vi "WMP Init.vi"(8 "error in (no error)":errorcluster, 11 "Main Panel in":refnum<class "Main Panel.lvclass">) -> (0 "error out":errorcluster, 3 "Main Panel out":refnum<class "Main Panel.lvclass">)   [LabVIEW 2018, in "Main Panel.lvlib" / "Main Panel.lvclass"]
uses:
  Main Panel.lvclass
  Main Panel.lvclass/Main Panel.ctl
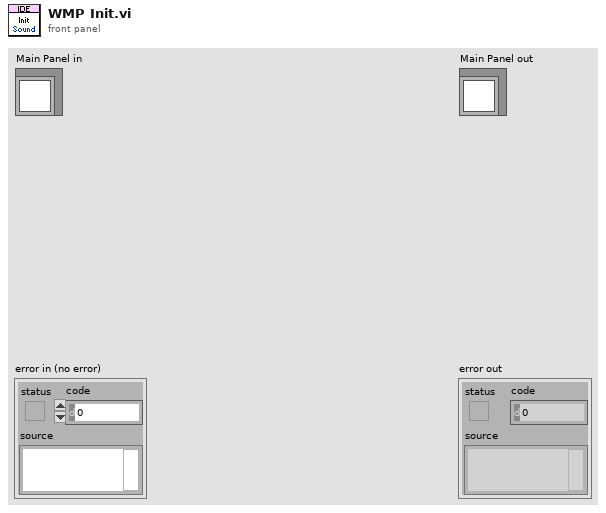
[diagram p1: front panel]
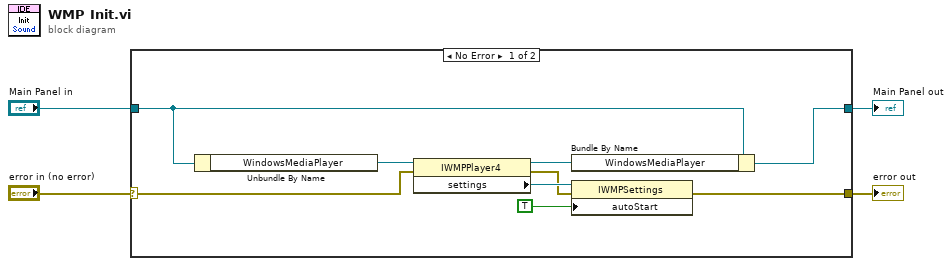
[diagram p0: block diagram]
diagram:
  n1 = case shown="No Error" "error in (no error)" {
    selector: "error in (no error)" -> [w8 w15]
    tunnel: [w7 w15] -> w3
    tunnel: [w6 w14] -> w1
    tunnel: "Main Panel in" -> [w10 w14]
    frame No Error {
      n2 = Unbundle By Name(w10) -> ("WindowsMediaPlayer"=w9:refnum<k7>)
      n3 = property class="IWMPPlayer4"(reference=w9, error in=w8) -> (reference out=w5:refnum<k7>, error out=w11:errorcluster, "settings"=w13:refnum<k7>)
      n4 = Bundle By Name(cluster=w10, "WindowsMediaPlayer"=w5) -> (w6:refnum<class "Main Panel.lvclass">)
      n5 = property class="IWMPSettings"(reference=w13, error in=w11, "autoStart"=TRUE) -> (error out=w7:errorcluster)  [unwired: 1 out]
    }
    frame Error {
    }
  }
  "error out" <- w3
  "Main Panel out" <- w1
